vi "b030写入合格信号.vi"(2 "信号":bool, 4 "产品ID":string) -> ()   [LabVIEW 2013]
uses:
  <vilib>/Utility/error.llb/whitespace.ctl
panel:
  in  "error in (no error)":errorcluster
  out "error out":errorcluster
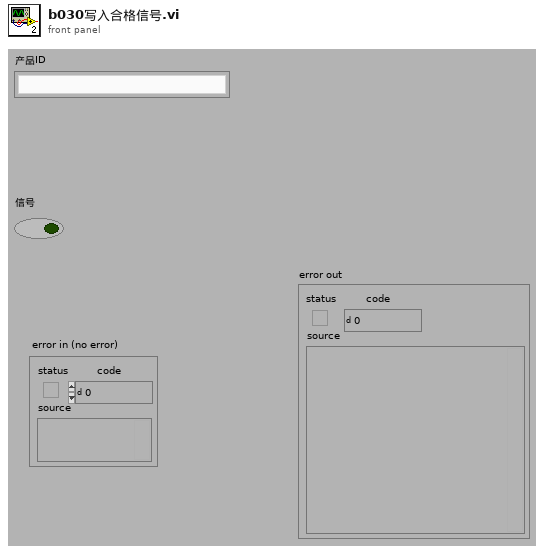
[diagram p1: front panel]
types:
  T1 = typedef "whitespace.ctl" = u16
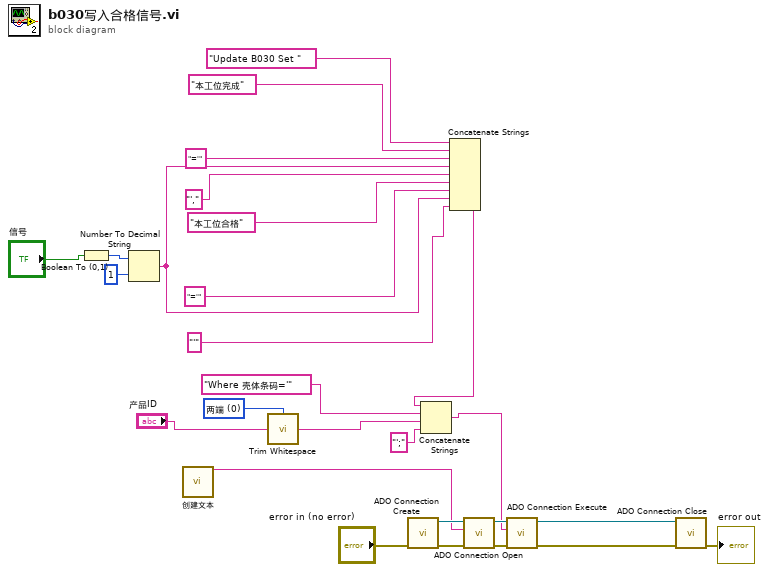
[diagram p0: block diagram]
diagram:
  w19 = T1 0 items=["两端", "字符串首端", "字符串末端"] ("location (both)")
  n1 = Boolean To (0,1)(Boolean="信号") -> (0, 1=w12:i16)
  n2 = Number To Decimal String(number=w12, width (-)=i16 1 ("宽度(-)")) -> (decimal integer string=w3:string)
  n3 = call "创建文本"() -> ("Result"=w15:string)  [unwired: 14 in, 1 out]
  n4 = call <vilib>:"Trim Whitespace.vi"("string"="产品ID", "location (both)"=w19) -> ("trimmed string"=w17:string)
  n5 = call "ADO Connection Create.vi"("error in (no error)"="error in (no error)") -> ("error out"=w26:errorcluster, "ADODB._Connection Out"=w27:refnum<k7>)  [unwired: 9 out]
  n6 = Concatenate Strings("Update B030 Set " ("字符串"), "本工位完成", "='", w3, "'," ("字符串"), "本工位合格", "='", w3, "'" ("字符串")) -> (w1:string)
  n7 = Concatenate Strings(w1, "Where 壳体条码='" ("字符串"), w17, "';" ("字符串")) -> (w14:string)
  n8 = call "ADO Connection Open.vi"("error in (no error)"=w26, "ConnectionString"=w15, "ADODB._Connection In"=w27) -> ("error out"=w25:errorcluster, "ADODB._Connection Out"=w24:refnum<k7>)  [unwired: 7 out]
  n9 = call "ADO Connection Execute.vi"("error in (no error)"=w25, "CommandText"=w14, "ADODB._Connection In"=w24) -> ("error out"=w20:errorcluster, "ADODB._Connection Out"=w23:refnum<k7>)  [unwired: 7 out]
  n10 = call "ADO Connection Close.vi"("error in (no error)"=w20, "ADODB._Connection In"=w23) -> ("error out"=→"error out":errorcluster)  [unwired: 9 out]
